vi "ManipWaitForPiece.vi"() -> (0 "Error Out":errorcluster, 1 "Advance Trigger":bool)   [LabVIEW 2023]
doc: "This VI pauses the manipulator sequencer until there is a note in the robot."
uses:
  GlobalNoteHandling.vi
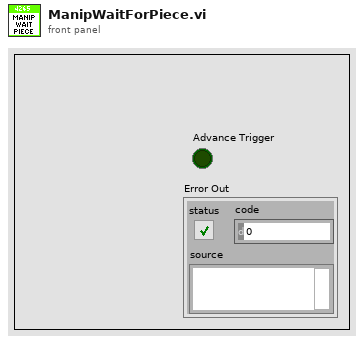
[diagram p1: front panel]
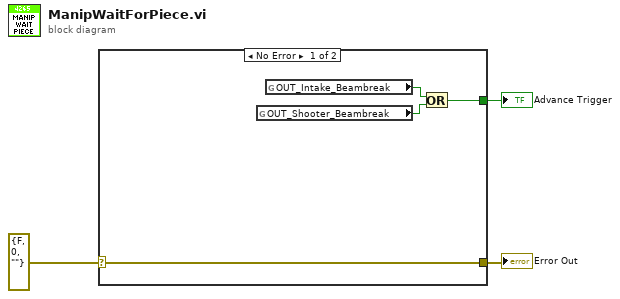
[diagram p0: block diagram]
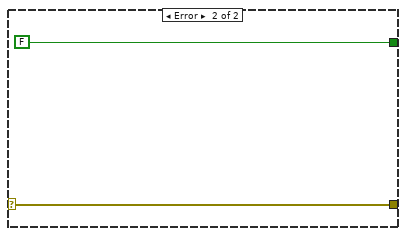
[diagram p2: hidden frame]
diagram:
  n1 = case shown="No Error" errorcluster {"status"=FALSE, "code"=0, "source"=""} ("error IO") {
    selector: errorcluster {"status"=FALSE, "code"=0, "source"=""} ("error IO") -> [w7 w9]
    tunnel: [w5 FALSE] -> w3
    tunnel: [w7 w9] -> w2
    frame No Error {
      n2 = global read "GlobalNoteHandling.vi" "OUT_Shooter_Beambreak"() -> (w6:bool)
      n3 = global read "GlobalNoteHandling.vi" "OUT_Intake_Beambreak"() -> (w4:bool)
      n4 = Or(x=w4, y=w6) -> (x .or. y?=w5:bool)
    }
    frame Error {
    }
  }
  "Advance Trigger" <- w3
  "Error Out" <- w2
